vi "GDC Kom.vi"(6 "Befehl":T3, 8 "error in (no error)":errorcluster caption="Fehler (Eingang, kein Fehler)", 10 "Daten":string[](array[string]), 11 "Serielle Parameter":T2={"VISA resource name"="", "timeout"=10000, "baud rate"=9600, "data bits "=8, "stop bits "=10, "Enable Termination\nChar (T)"=TRUE, "termination char\n(0xA = '\\n' = LF) "=13} {"termination char\n(0xA = '\\n' = LF)" format="%.0x"; "stop bits" items=["1.0"=10, "1.5"=15, "2.0"=20]; "data bits" min=5 max=8 step=1}) -> (0 "error out":errorcluster caption="Fehler (Ausgang)", 1 "Status (alarm)":bool, 2 "Gas":string[](array[string]), 3 "Fehler":bool, 4 "Status":string, 5 "Konzentration":string, 7 "Konzentration 2":string)   [LabVIEW 2020, in "Linearisierung v2.lvlib" / "Gasteiler.lvlib" / "Horiba GDC.lvlib"]
uses:
  Horiba GDC.lvlib
  Aktion Befehl.ctl
  Serielle Parameter.ctl
  Stats.ctl
  Aktionen FGV Gasteiler Daten.ctl
  <vilib>/Instr/_visa.llb/VISA Configure Serial Port (Instr).vi
  Gasteiler.lvlib
panel:
  out "Status":T1
  out "Daten":string
  out "Befehl":string
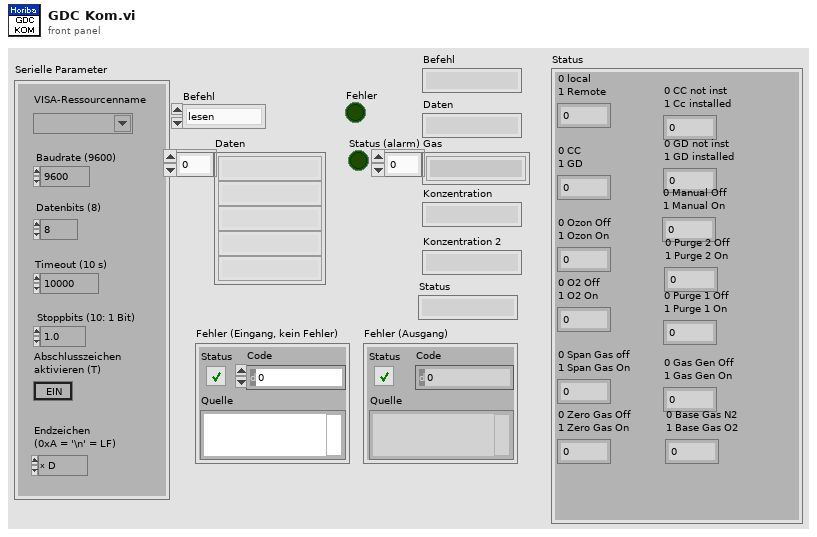
[diagram p1: front panel]
types:
  T1 = typedef "Linearisierung v2.lvlib/Gasteiler.lvlib/Horiba GDC.lvlib/Stats.ctl" = cluster{"0 local\n1 Remote":i16, "0 CC\n1 GD":i16, "0 Ozon Off\n1 Ozon On":i16, "0 O2 Off\n1 O2 On":i16, "0 Span Gas off\n1 Span Gas On ":i16, "0 Zero Gas Off\n1 Zero Gas On":i16, "0 CC not inst\n1 Cc installed":i16, "0 GD not inst\n1 GD installed":i16, "0 Manual Off\n1 Manual On":i16, "0 Purge 2 Off\n1 Purge 2 On":i16, "0 Purge 1 Off\n1 Purge 1 On":i16, "0 Gas Gen Off\n1 Gas Gen On":i16, "0 Base Gas N2\n1 Base Gas O2":i16}
  T2 = typedef "Linearisierung v2.lvlib/Gasteiler.lvlib/Horiba GDC.lvlib/Serielle Parameter.ctl" = cluster{"VISA resource name":refnum<visa-resource-name>, "timeout":u32, "baud rate":u32, "data bits ":u16, "stop bits ":u16, "Enable Termination\nChar (T)":bool, "termination char\n(0xA = '\\n' = LF) ":u8}
  T3 = typedef "Linearisierung v2.lvlib/Gasteiler.lvlib/Horiba GDC.lvlib/Aktion Befehl.ctl" = enum16{"lesen", "initialisieren", "Beenden", "Standby", "GD/CC", "Info", "Flow", "Alarm", "GD parameter", "GD point", "Durchfluss", "Spuelen1", "Spuelen1 On", "Spuelen1Off", "Spuelen2", "Ventil-Abfrage", "Reset"}
  T4 = typedef "Linearisierung v2.lvlib/Gasteiler.lvlib/Aktionen FGV Gasteiler Daten.ctl" = enum16{"lesen", "Gasteiler Daten", "Seriellen Param.", "MB-Endwert", "laden", "speichern", "Anforderung", "TCP", "Aufzeichnung Start"}
  T5 = typedef "AK-Schnittstelle.lvlib/AK Seriell.lvlib/Serielle Parameter.ctl" = cluster{"VISA resource name":refnum<visa-resource-name>, "baud rate":u32, "data bits":u16, "parity":u16, "stop bits":u16, "flow control":u16}
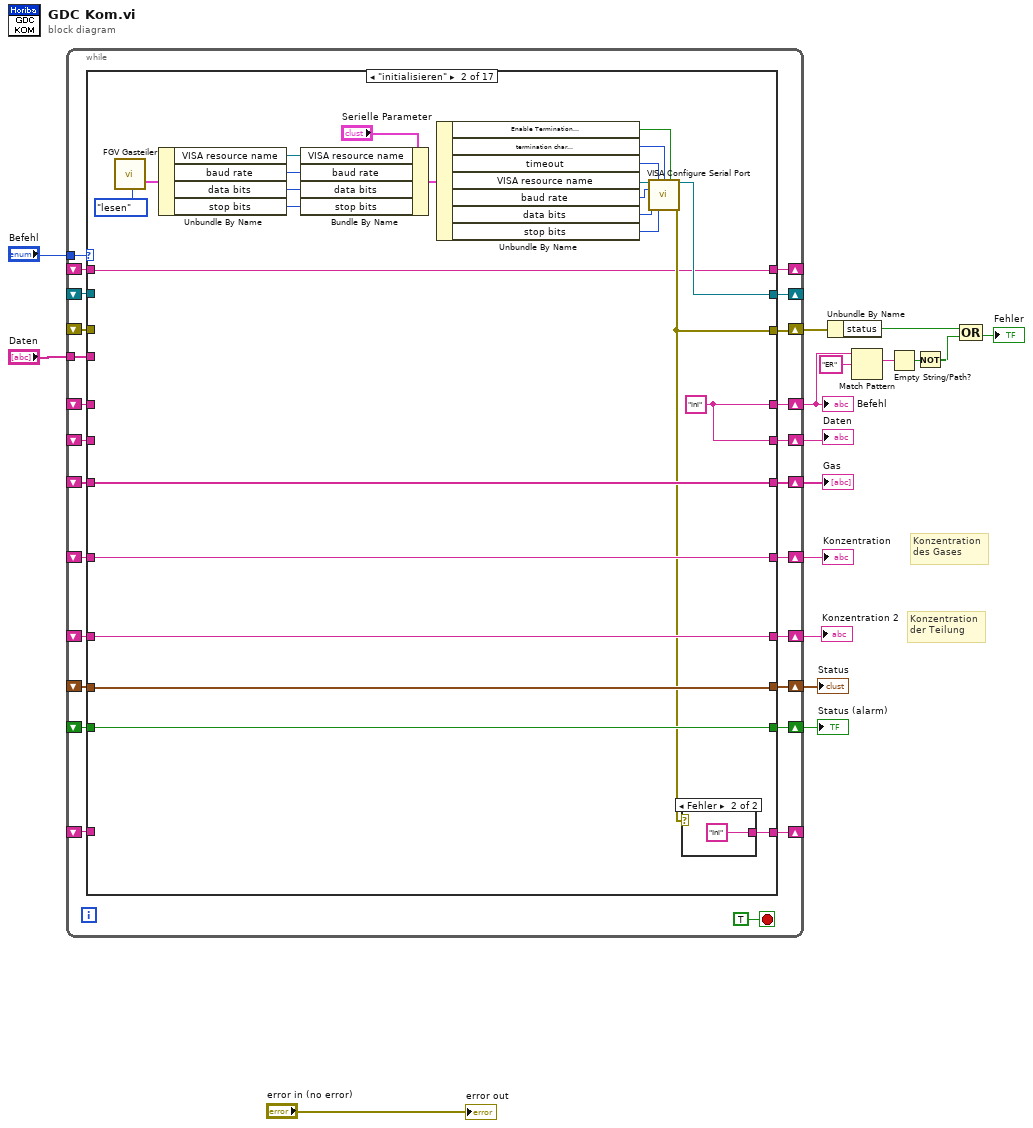
[diagram p0: block diagram]
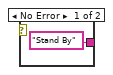
[diagram p3: hidden frame]
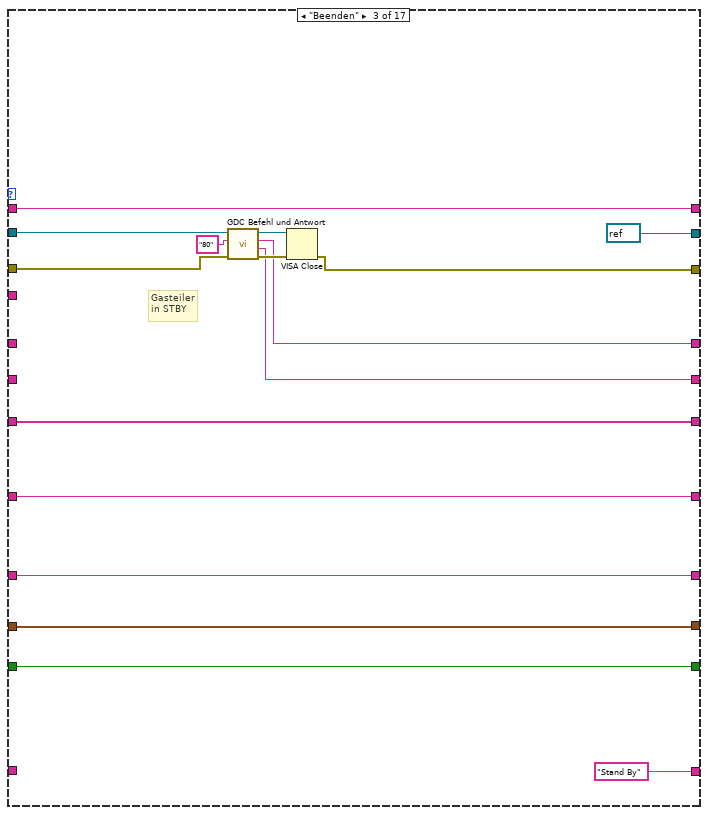
[diagram p4: hidden frame]
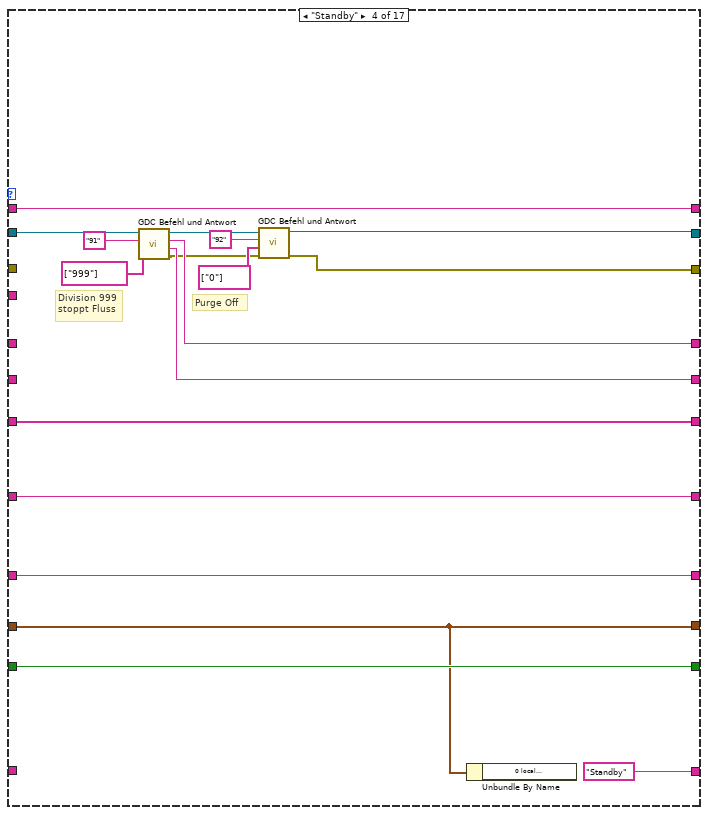
[diagram p5: hidden frame]
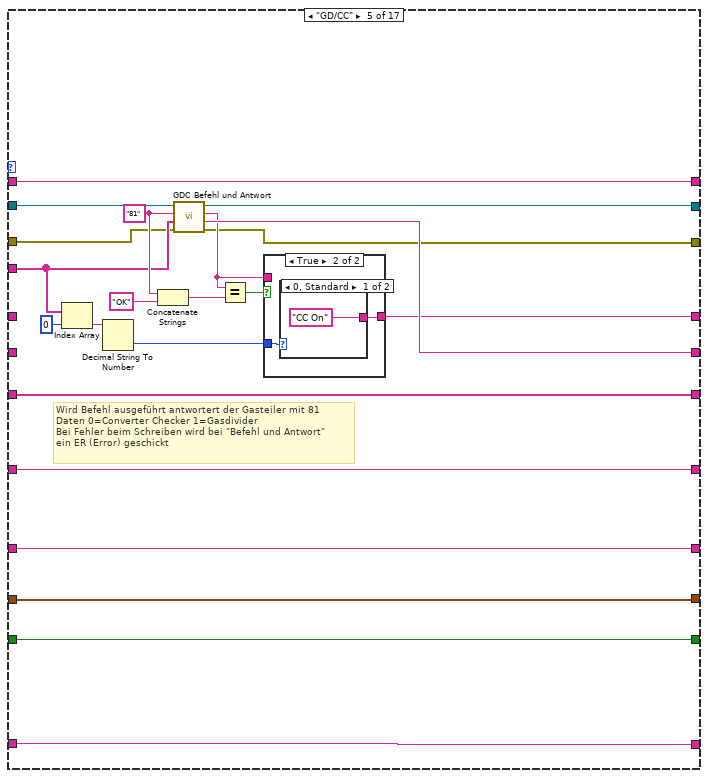
[diagram p6: hidden frame]
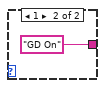
[diagram p8: hidden frame]
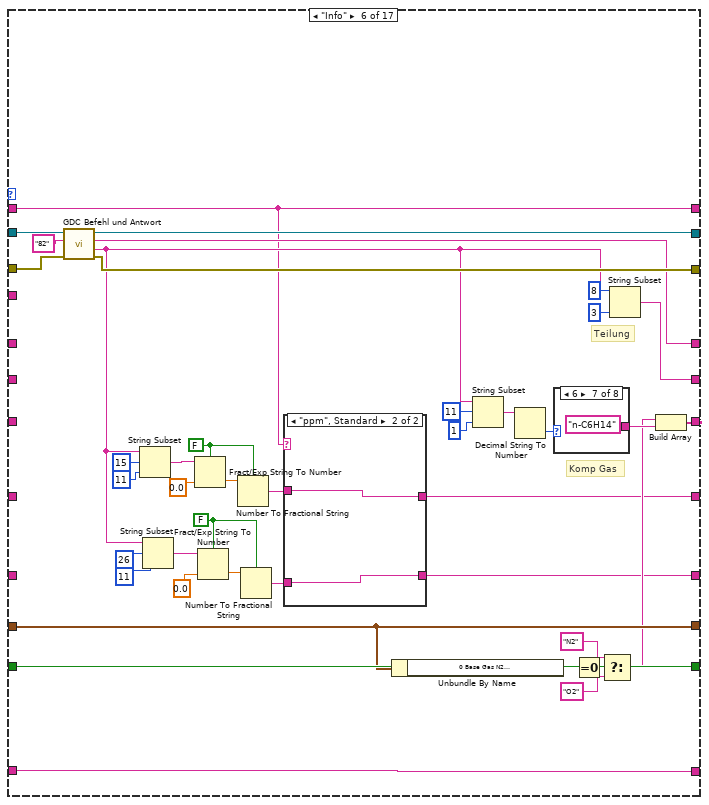
[diagram p9: hidden frame]
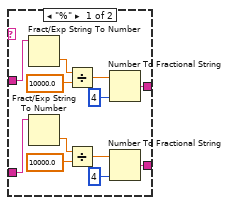
[diagram p10: hidden frame]
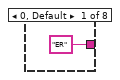
[diagram p11: hidden frame]
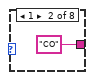
[diagram p12: hidden frame]
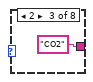
[diagram p13: hidden frame]
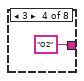
[diagram p14: hidden frame]
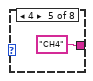
[diagram p15: hidden frame]
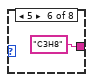
[diagram p16: hidden frame]
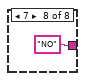
[diagram p17: hidden frame]
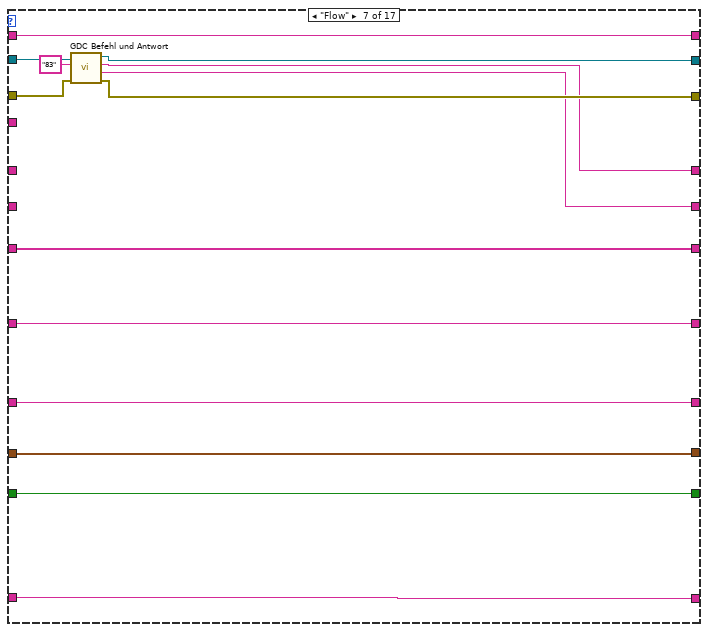
[diagram p18: hidden frame]
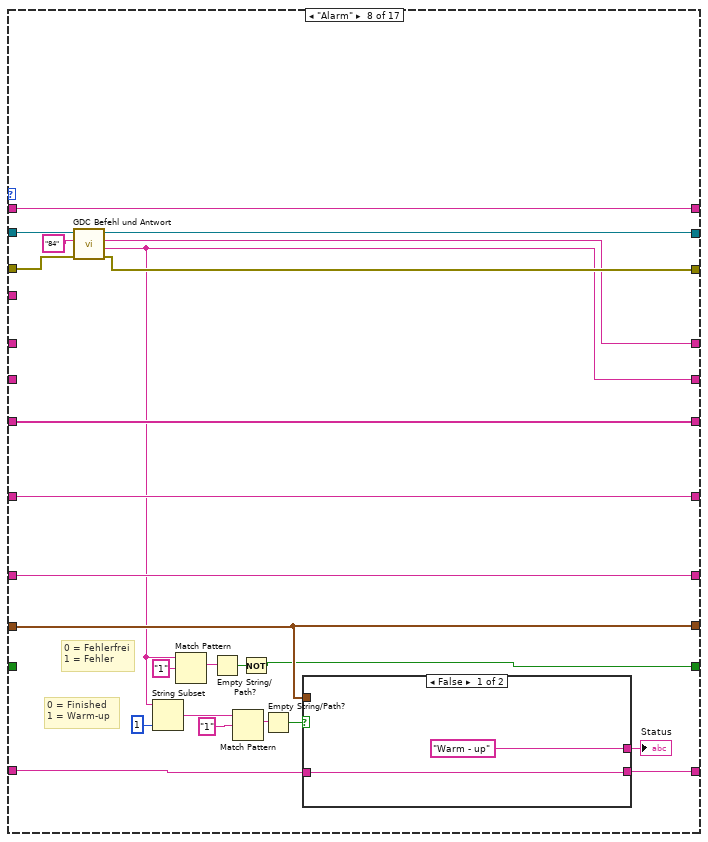
[diagram p19: hidden frame]
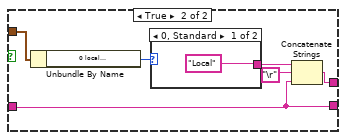
[diagram p20: hidden frame]
diagram:
  # "Konzentration\nder Teilung"
  # "Konzentration\ndes Gases"
  n1 = while {
    tunnel: "Befehl" -> [w41]
    shift-right: [w40] -> _
    shift-left: _ -> [w39]
    shift-right: [w38] -> w3
    shift-left: _ -> [w37]
    tunnel: "Daten" -> [w35]
    shift-right: [w36] -> w8
    shift-left: _ -> [w29]
    shift-right: [w34] -> w15
    shift-left: _ -> [w28]
    shift-right: [w33] -> w14
    shift-left: _ -> [w27]
    shift-right: [w32] -> w13
    shift-left: _ -> [w26]
    shift-right: [w31] -> w12
    shift-left: _ -> [w25]
    shift-right: [w30] -> w4
    shift-left: _ -> [w24]
    shift-right: [w23] -> w2
    shift-left: _ -> [w22]
    shift-right: [w20] -> _
    shift-left: _ -> [w21]
    shift-right: [w19] -> _
    shift-left: _ -> [w18]
    stop <- TRUE stop-if-true
    n2 = case shown="\"initialisieren\"" w41 {
      tunnel: [w53 w73 refnum<visa-resource-name> refnum ("VISA resource name out") w100 w135 w180 w209 w238 w285 w309 w371 w386 w401 w414 w425 w439 w453] -> w40
      tunnel: w39 -> [w53 _ w91 w114 w136 w182 w213 w242 w288 w334 w373 w388 w403 w417 w429 w441 w455]
      tunnel: [w52 w56 w95 w101 w124 w179 w210 w239 w284 w307 w370 w385 w400 w413 w424 w440 w452] -> w38
      tunnel: w37 -> [w52 _ w92 _ w125 w181 w211 w241 w287 w333 w372 w387 w402 w416 w428 w442 w454]
      tunnel: [w51 w72 w85 w112 w131 w158 w208 w232 w283 w308 w367 w383 w398 w412 w423 w438 w451] -> w36
      tunnel: w35 -> [_ _ _ _ w129 _ _ _ w257 w331 w368 _ _ w415 _ _ _]
      tunnel: [w50 w72 w84 w111 w134 w176 w207 w220 w282 w306 w366 w382 w397 w411 w422 w437 w461] -> w34
      tunnel: [w49 w71 w90 w110 w123 w154 w218 w222 w281 w302 w365 w381 w396 w410 w433 w447 w460] -> w33
      tunnel: [w48 w70 w89 w109 w122 w143 w217 w234 w261 w292 w364 w380 w395 w409 w432 w446 w459] -> w32
      tunnel: [w47 w69 w88 w108 w121 w142 w216 w233 w280 w291 w363 w379 w394 w408 w431 w445 w458] -> w31
      tunnel: [w46 w68 w87 w107 w120 w157 w215 w219 w279 w330 w362 w378 w393 w407 w430 w444 w457] -> w30
      tunnel: w29 -> [w51 _ _ _ _ _ _ _ _ _ _ _ _ _ _ _ _]
      tunnel: w28 -> [w50 _ _ _ _ _ _ _ _ _ _ _ _ _ _ _ w461]
      tunnel: w27 -> [w49 w71 w90 w110 w123 _ w218 w222 w281 _ w365 w381 w396 w410 w433 w447 w460]
      tunnel: w26 -> [w48 w70 w89 w109 w122 _ w217 w234 w261 _ w364 w380 w395 w409 w432 w446 w459]
      tunnel: w25 -> [w47 w69 w88 w108 w121 _ w216 w233 w280 _ w363 w379 w394 w408 w431 w445 w458]
      tunnel: w24 -> [w46 w68 w87 w107 w120 w157 w215 _ w279 w330 w362 w378 w393 w407 w430 w444 w457]
      tunnel: [w45 w58 w83 w99 w117 w149 w214 w223 w260 w296 w361 w377 w392 w406 w421 w436 w450] -> w23
      tunnel: w22 -> [w45 w58 w83 w99 w117 w149 w214 w223 w260 _ w361 w377 w392 w406 w421 w436 w450]
      tunnel: w21 -> [w44 _ _ _ w116 w155 w206 w226 _ _ _ _ _ _ w420 w435 _]
      tunnel: [w44 w57 "Stand By" "Standby" w116 w155 w206 w225 "Set" "CalGas" "Purge" "Purge" "Stand By" "Purge Air" w420 w435 "Stand By"] -> w20
      tunnel: [w43 w55 w81 w97 w115 w144 w205 w221 w254 w293 w359 w374 w389 w404 w419 w434 w448] -> w19
      tunnel: w18 -> [w43 w55 w81 w97 w115 w144 w205 w221 _ w293 w359 w374 w389 w404 w419 w434 w448]
      frame "lesen", Default {
      }
      frame "initialisieren" {
        w72 = "ini" ("Befehl")
        n3 = call "FGV Gasteiler.vi"("Aktionen"=Aktionen_FGV_Gasteiler_Daten."lesen") -> ("Serielle Parameter"=w65:T5)  [unwired: 11 in, 7 out]
        n4 = Unbundle By Name(w65) -> ("VISA resource name"=w59:refnum<visa-resource-name>, "baud rate"=w60:u32, "data bits"=w61:u16, "stop bits"=w62:u16)
        n5 = Bundle By Name(cluster="Serielle Parameter", "VISA resource name"=w59, "baud rate"=w60, "data bits"=w61, "stop bits"=w62) -> (w64:T2)
        n6 = Unbundle By Name(w64) -> ("Enable Termination\nChar (T)"=w67:bool, "termination char\n(0xA = '\\n' = LF)"=w66:u8, "timeout"=w78:u32, "VISA resource name"=w77:refnum<visa-resource-name>, "baud rate"=w76:u32, "data bits"=w75:u16, "stop bits"=w74:u16)
        n7 = call-poly "VISA Configure Serial Port"("VISA resource name"=w77, "timeout (10sec)"=w78, "termination char\n(0xA = '\\n' = LF)"=w66, "Enable Termination\nChar (T)"=w67, "baud rate (9600)"=w76, "data bits (8)"=w75, "stop bits (10: 1 bit)"=w74) -> ("VISA resource name out"=w73:refnum<visa-resource-name>, "error out"=w56:errorcluster)  [unwired: 7 in]
        n8 = case shown="Fehler" w56 {
          tunnel: ["Stand By" "Ini" ("Befehl")] -> w57
          frame No Error {
          }
          frame Error {
          }
        }
      }
      frame "Beenden" {
        # "Gasteiler\nin STBY"
        n9 = call "GDC Befehl und Antwort.vi"("error in (no error)"=w92, "Befehl"="80", "VISA-Ressourcenname"=w91) -> ("error out"=w93:errorcluster, "Daten"=w84:string, "Befehl"=w85:string, "VISA-Ressourcenname (Ausgang)"=w86:refnum<visa-resource-name>)  [unwired: 5 in]
        n10 = VISA Close(VISA resource name=w86, error in (no error)=w93) -> (error out=w95:errorcluster)
      }
      frame "Standby" {
        # "Purge Off"
        # "Division 999\nstoppt Fluss"
        n11 = call "GDC Befehl und Antwort.vi"("Daten"=string[] ["999"], "Befehl"="91", "VISA-Ressourcenname"=w114) -> ("error out"=w102:errorcluster, "Daten"=w111:string, "Befehl"=w112:string, "VISA-Ressourcenname (Ausgang)"=w103:refnum<visa-resource-name>)  [unwired: 5 in]
        n12 = call "GDC Befehl und Antwort.vi"("error in (no error)"=w102, "Daten"=string[] ["0"], "Befehl"="92", "VISA-Ressourcenname"=w103) -> ("error out"=w101:errorcluster, "VISA-Ressourcenname (Ausgang)"=w100:refnum<visa-resource-name>)  [unwired: 4 in, 2 out]
        n13 = Unbundle By Name(w99) -> ()  [unwired: 1 out]
      }
      frame "GD/CC" {
        w133 = "81" ("Befehl")
        # "Wird Befehl ausgeführt antwortert der Gasteiler mit 81\nDaten 0=Converter Checker 1=Gasdivider\nBei Fehler beim Schreiben wird bei \"Befehl und Antwort\"\nein ER (Error) geschickt"
        n14 = Index Array(array=w129, index=0 ("Index")) -> (element=w127:string)
        n15 = Decimal String To Number(string=w127) -> (number=w126:i32)  [unwired: 2 in, 1 out]
        n16 = Concatenate Strings(w133, "OK" ("String")) -> (w119:string)
        n17 = call "GDC Befehl und Antwort.vi"("error in (no error)"=w125, "Daten"=w129, "Befehl"=w133, "VISA-Ressourcenname"=w136) -> ("error out"=w124:errorcluster, "Daten"=w134:string, "Befehl"=w130:string, "VISA-Ressourcenname (Ausgang)"=w135:refnum<visa-resource-name>)  [unwired: 4 in]
        n18 = Equal?(x=w130, y=w119) -> (x = y?=w132:bool)
        n19 = case shown="True" w132 {
          tunnel: [w137 w138] -> w131
          tunnel: w130 -> [w137 _]
          tunnel: w126 -> [_ w139]
          frame False {
          }
          frame True {
            n20 = case shown="0, Standard" w139 {
              tunnel: ["CC On" ("Befehl") "GD On" ("Befehl")] -> w138
              frame 0, Default {
              }
              frame 1 {
              }
            }
          }
        }
      }
      frame "Info" {
        w165 = FALSE ("Systemdezimalzeichen verwenden (T)")
        w166 = FALSE ("Systemdezimalzeichen verwenden (T)")
        # "Komp Gas"
        # "Teilung"
        n21 = call "GDC Befehl und Antwort.vi"("error in (no error)"=w181, "Befehl"="82", "VISA-Ressourcenname"=w182) -> ("error out"=w179:errorcluster, "Daten"=w159:string, "Befehl"=w158:string, "VISA-Ressourcenname (Ausgang)"=w180:refnum<visa-resource-name>)  [unwired: 5 in]
        n22 = String Subset(string=w159, offset (0)=15 ("Offset (0)"), length (rest)=11 ("Länge (Rest)")) -> (substring=w169:string)
        n23 = String Subset(string=w159, offset (0)=26 ("Offset (0)"), length (rest)=11 ("Länge (Rest)")) -> (substring=w162:string)
        n24 = Fract/Exp String To Number(use system decimal point (T)=w166, string=w169, default (0 dbl)=sgl 0.0 ("Standard (0 DBL)")) -> (number=w167:sgl)  [unwired: 1 in, 1 out]
        n25 = Fract/Exp String To Number(use system decimal point (T)=w165, string=w162, default (0 dbl)=sgl 0.0 ("Standard (0 DBL)")) -> (number=w164:sgl)  [unwired: 1 in, 1 out]
        n26 = Number To Fractional String(use system decimal point (T)=w166, number=w167) -> (F-format string=w146:string)  [unwired: 2 in]
        n27 = Number To Fractional String(use system decimal point (T)=w165, number=w164) -> (F-format string=w145:string)  [unwired: 2 in]
        n28 = case shown="\"ppm\", Standard" w144 {
          tunnel: [w190 w195] -> w142
          tunnel: [w185 w196] -> w143
          tunnel: w146 -> [w184 w196]
          tunnel: w145 -> [w183 w195]
          frame "%" {
            n29 = Fract/Exp String To Number(string=w184) -> (number=w187:dbl)  [unwired: 3 in, 1 out]
            n30 = Fract/Exp String To Number(string=w183) -> (number=w193:dbl)  [unwired: 3 in, 1 out]
            n31 = Divide(x=w187, y=10000.0) -> (x/y=w188:dbl)
            n32 = Divide(x=w193, y=10000.0) -> (x/y=w192:dbl)
            n33 = Number To Fractional String(number=w188, precision (6)=i16 4 ("Genauigkeit (6)")) -> (F-format string=w185:string)  [unwired: 2 in]
            n34 = Number To Fractional String(number=w192, precision (6)=i16 4 ("Genauigkeit (6)")) -> (F-format string=w190:string)  [unwired: 2 in]
          }
          frame "ppm", Default {
          }
        }
        n35 = Unbundle By Name(w149) -> ("0 Base Gas N2\n1 Base Gas O2"=w153:i16)
        n36 = String Subset(string=w159, offset (0)=11 ("Offset (0)"), length (rest)=1 ("Länge (Rest)")) -> (substring=w173:string)
        n37 = Decimal String To Number(string=w173) -> (number=w172:i32)  [unwired: 2 in, 1 out]
        n38 = case shown="6" w172 {
          tunnel: ["ER" ("Befehl") "CO" ("Befehl") "CO2" ("Befehl") "O2" ("Befehl") "CH4" ("Befehl") "C3H8" ("Befehl") "n-C6H14" ("Befehl") "NO" ("Befehl")] -> w148
          frame 0, Default {
          }
          frame 1 {
          }
          frame 2 {
          }
          frame 3 {
          }
          frame 4 {
          }
          frame 5 {
          }
          frame 6 {
          }
          frame 7 {
          }
        }
        n39 = Equal To 0?(x=w153) -> (x = 0?=w151:bool)
        n40 = Select(t="N2", s=w151, f="O2") -> (s? t:f=w147:string)
        n41 = String Subset(string=w159, offset (0)=8 ("Offset (0)"), length (rest)=3 ("Länge (Rest)")) -> (substring=w176:string)
        n42 = Build Array(w147, w148) -> (w154:string[])
      }
      frame "Flow" {
        n43 = call "GDC Befehl und Antwort.vi"("error in (no error)"=w211, "Befehl"="83", "VISA-Ressourcenname"=w213) -> ("error out"=w210:errorcluster, "Daten"=w207:string, "Befehl"=w208:string, "VISA-Ressourcenname (Ausgang)"=w209:refnum<visa-resource-name>)  [unwired: 5 in]
      }
      frame "Alarm" {
        # "0 = Finished\n1 = Warm-up"
        # "0 = Fehlerfrei\n1 = Fehler"
        n44 = call "GDC Befehl und Antwort.vi"("error in (no error)"=w241, "Befehl"="84", "VISA-Ressourcenname"=w242) -> ("error out"=w239:errorcluster, "Daten"=w220:string, "Befehl"=w232:string, "VISA-Ressourcenname (Ausgang)"=w238:refnum<visa-resource-name>)  [unwired: 5 in]
        n45 = String Subset(string=w220, length (rest)=1 ("Länge (Rest)")) -> (substring=w228:string)  [unwired: 1 in]
        n46 = Match Pattern(string=w220, regular expression="1" ("Regulärer Ausdruck")) -> (match substring=w236:string)  [unwired: 1 in, 3 out]
        n47 = Empty String/Path?(string/path=w236) -> (empty?=w235:bool)
        n48 = Match Pattern(string=w228, regular expression="1" ("Regulärer Ausdruck")) -> (match substring=w230:string)  [unwired: 1 in, 3 out]
        n49 = Not(x=w235) -> (.not. x?=w219:bool)
        n50 = Empty String/Path?(string/path=w230) -> (empty?=w227:bool)
        n51 = case shown="False" w227 {
          tunnel: w223 -> [_ w250]
          tunnel: ["Warm - up" w248] -> w224
          tunnel: w226 -> [w243 w246]
          tunnel: [w243 w246] -> w225
          frame False {
          }
          frame True {
            n52 = Unbundle By Name(w250) -> ("0 local\n1 Remote"=w249:i16)
            n53 = case shown="0, Standard" w249 {
              tunnel: ["Local" ("Regulärer Ausdruck") "Remote" ("Regulärer Ausdruck")] -> w247
              frame 0, Default {
              }
              frame 1 {
              }
            }
            n54 = Concatenate Strings(w247, "\r", w246) -> (w248:string)
          }
        }
        "Status" <- w224
      }
      frame "GD parameter" {
        # "#GenauSysFix"
        # "Befehl:\n90\nx - 1-7 für Komp Gas\nx - 1-2 für Träger Gas\nxxx - Teilung (z.B. 001 -500)\nxxxxxxxxxxx - für Konzentration in ppm z.B. +1.23456E+09"
        n55 = Array Size(array=w257) -> (size(s)=w258:i32)
        n56 = Decrement(x=w258) -> (x-1=w256:i32)
        n57 = Delete From Array(array=w257, index=w256) -> (deleted portion=w254:string, array with subset deleted=w255:string[])  [unwired: 1 in]
        n58 = Index Array(array=w255, index=3 ("Index")) -> (element=w272:string)
        n59 = Fract/Exp String To Number(use system decimal point (T)=FALSE ("Systemdezimalzeichen verwenden (T)"), string=w272, default (0 dbl)=sgl 0.0 ("Standard (0 I32)")) -> (number=w276:sgl)  [unwired: 1 in, 1 out]
        n60 = Number To Exponential String(number=w276, precision (6)=i16 4 ("Genauigkeit (6)"), 1:FALSE ("Systemdezimalzeichen verwenden (T)")) -> (E-format string=w266:string)  [unwired: 1 in]
        n61 = String Subset(string=w266, length (rest)=8 ("Länge (Rest)")) -> (substring=w263:string)  [unwired: 1 in]
        n62 = String Subset(string=w266, offset (0)=8 ("Offset (0)")) -> (substring=w267:string)  [unwired: 1 in]
        n63 = Concatenate Strings(w263, "0" ("String"), w267) -> (w265:string)
        n64 = Concatenate Strings("+" ("String"), w265) -> (w271:string)
        n65 = Replace Array Subset(array=w255, new element=w271, index=3 ("Index")) -> (w273:string[])
        n66 = call "GDC Befehl und Antwort.vi"("error in (no error)"=w287, "Daten"=w273, "Befehl"="90", "VISA-Ressourcenname"=w288) -> ("error out"=w284:errorcluster, "Daten"=w282:string, "Befehl"=w283:string, "VISA-Ressourcenname (Ausgang)"=w285:refnum<visa-resource-name>)  [unwired: 4 in]
      }
      frame "GD point" {
        w317 = FALSE ("Systemdezimalzeichen verwenden (T)")
        w318 = FALSE ("Systemdezimalzeichen verwenden (T)")
        # "Konzentration des \naktuellen Punkts\nund Konzentration \ndes Gases???"
        # "Komp Gas"
        # "Teilung"
        # "Befehl\n91\nxxx - Teilungsstufe z.B. 192"
        n67 = call "GDC Befehl und Antwort.vi"("error in (no error)"=w333, "Daten"=w331, "Befehl"="91", "VISA-Ressourcenname"=w334) -> ("error out"=w290:errorcluster, "VISA-Ressourcenname (Ausgang)"=w310:refnum<visa-resource-name>)  [unwired: 4 in, 2 out]
        n68 = flat-sequence {
          tunnel: w290 -> [w335]
          tunnel: [w335] -> w289
          frame #0 {
            n69 = Wait (ms)(milliseconds to wait=u32 500 ("Zu wartende ms")) -> ()  [unwired: 1 out]
          }
        }
        n70 = call "GDC Befehl und Antwort.vi"("error in (no error)"=w289, "Befehl"="82", "VISA-Ressourcenname"=w310) -> ("error out"=w307:errorcluster, "Daten"=w304:string, "Befehl"=w308:string, "VISA-Ressourcenname (Ausgang)"=w309:refnum<visa-resource-name>)  [unwired: 5 in]
        n71 = call "Hex String.vi"("Eingabe String"=w304) -> ("Status"=w296:T1)  [unwired: 10 in]
        n72 = String Subset(string=w304, offset (0)=26 ("Offset (0)"), length (rest)=11 ("Länge (Rest)")) -> (substring=w314:string)
        n73 = String Subset(string=w304, offset (0)=15 ("Offset (0)"), length (rest)=11 ("Länge (Rest)")) -> (substring=w321:string)
        n74 = Unbundle By Name(w296) -> ("0 Base Gas N2\n1 Base Gas O2"=w301:i16)
        n75 = Fract/Exp String To Number(use system decimal point (T)=w317, string=w314, default (0 dbl)=sgl 0.0 ("Standard (0 DBL)")) -> (number=w316:sgl)  [unwired: 1 in, 1 out]
        n76 = Fract/Exp String To Number(use system decimal point (T)=w318, string=w321, default (0 dbl)=sgl 0.0 ("Standard (0 DBL)")) -> (number=w319:sgl)  [unwired: 1 in, 1 out]
        n77 = Number To Fractional String(use system decimal point (T)=w317, number=w316) -> (F-format string=w294:string)  [unwired: 2 in]
        n78 = Number To Fractional String(use system decimal point (T)=w318, number=w319) -> (F-format string=w295:string)  [unwired: 2 in]
        n79 = case shown="\"ppm\", Standard" w293 {
          tunnel: [w344 w349] -> w291
          tunnel: [w339 w350] -> w292
          tunnel: w295 -> [w338 w350]
          tunnel: w294 -> [w337 w349]
          frame "%" {
            n80 = Fract/Exp String To Number(string=w338) -> (number=w341:dbl)  [unwired: 3 in, 1 out]
            n81 = Fract/Exp String To Number(string=w337) -> (number=w347:dbl)  [unwired: 3 in, 1 out]
            n82 = Divide(x=w341, y=10000.0) -> (x/y=w342:dbl)
            n83 = Divide(x=w347, y=10000.0) -> (x/y=w346:dbl)
            n84 = Number To Fractional String(number=w342, precision (6)=i16 4 ("Genauigkeit (6)")) -> (F-format string=w339:string)  [unwired: 2 in]
            n85 = Number To Fractional String(number=w346, precision (6)=i16 4 ("Genauigkeit (6)")) -> (F-format string=w344:string)  [unwired: 2 in]
          }
          frame "ppm", Default {
          }
        }
        n86 = String Subset(string=w304, offset (0)=11 ("Offset (0)"), length (rest)=1 ("Länge (Rest)")) -> (substring=w325:string)
        n87 = Decimal String To Number(string=w325) -> (number=w324:i32)  [unwired: 2 in, 1 out]
        n88 = Equal To 0?(x=w301) -> (x = 0?=w299:bool)
        n89 = Select(t="N2", s=w299, f="O2") -> (s? t:f=w297:string)
        n90 = case shown="0, Standard" w324 {
          tunnel: ["ER" ("Befehl") "CO" ("Befehl") "CO2" ("Befehl") "O2" ("Befehl") "CH4" ("Befehl") "C3H8" ("Befehl") "n-C6H14" ("Befehl") "NO" ("Befehl")] -> w305
          frame 0, Default {
          }
          frame 1 {
          }
          frame 2 {
          }
          frame 3 {
          }
          frame 4 {
          }
          frame 5 {
          }
          frame 6 {
          }
          frame 7 {
          }
        }
        n91 = String Subset(string=w304, offset (0)=8 ("Offset (0)"), length (rest)=3 ("Länge (Rest)")) -> (substring=w306:string)
        n92 = Build Array(w297, w305) -> (w302:string[])
      }
      frame "Spuelen1" {
        # "Purge 1 für GD\n0 = Reset\n1 = Purge"
        n93 = call "GDC Befehl und Antwort.vi"("error in (no error)"=w372, "Daten"=w368, "Befehl"="92", "VISA-Ressourcenname"=w373) -> ("error out"=w370:errorcluster, "Daten"=w366:string, "Befehl"=w367:string, "VISA-Ressourcenname (Ausgang)"=w371:refnum<visa-resource-name>)  [unwired: 4 in]
      }
      frame "Spuelen1 On" {
        # "Purge 1 für GD\n0 = Reset\n1 = Purge"
        n94 = call "GDC Befehl und Antwort.vi"("error in (no error)"=w387, "Daten"=string[] ["1"], "Befehl"="92", "VISA-Ressourcenname"=w388) -> ("error out"=w385:errorcluster, "Daten"=w382:string, "Befehl"=w383:string, "VISA-Ressourcenname (Ausgang)"=w386:refnum<visa-resource-name>)  [unwired: 4 in]
      }
      frame "Spuelen1Off" {
        # "Purge 1 für GD\n0 = Reset\n1 = Purge"
        n95 = call "GDC Befehl und Antwort.vi"("error in (no error)"=w402, "Daten"=string[] ["0"], "Befehl"="92", "VISA-Ressourcenname"=w403) -> ("error out"=w400:errorcluster, "Daten"=w397:string, "Befehl"=w398:string, "VISA-Ressourcenname (Ausgang)"=w401:refnum<visa-resource-name>)  [unwired: 4 in]
      }
      frame "Spuelen2" {
        # "Purge 2 für GD\n0 = Reset\n1 = Purge"
        n96 = call "GDC Befehl und Antwort.vi"("error in (no error)"=w416, "Daten"=w415, "Befehl"="93", "VISA-Ressourcenname"=w417) -> ("error out"=w413:errorcluster, "Daten"=w411:string, "Befehl"=w412:string, "VISA-Ressourcenname (Ausgang)"=w414:refnum<visa-resource-name>)  [unwired: 4 in]
      }
      frame "Durchfluss" {
        # "NO Konz"
        # "Span Gas"
        # "Zero Gas"
        n97 = call "GDC Befehl und Antwort.vi"("error in (no error)"=w428, "Daten"=string[] ["0000", "4000", "0000000000"], "Befehl"="BD", "VISA-Ressourcenname"=w429) -> ("error out"=w424:errorcluster, "Daten"=w422:string, "Befehl"=w423:string, "VISA-Ressourcenname (Ausgang)"=w425:refnum<visa-resource-name>)  [unwired: 4 in]
      }
      frame "Ventil-Abfrage" {
        n98 = call "GDC Befehl und Antwort.vi"("error in (no error)"=w442, "Befehl"="B7", "VISA-Ressourcenname"=w441) -> ("error out"=w440:errorcluster, "Daten"=w437:string, "Befehl"=w438:string, "VISA-Ressourcenname (Ausgang)"=w439:refnum<visa-resource-name>)  [unwired: 5 in]
      }
      frame "Reset" {
        n99 = call "GDC Befehl und Antwort.vi"("error in (no error)"=w454, "Befehl"="80", "VISA-Ressourcenname"=w455) -> ("error out"=w452:errorcluster, "Befehl"=w451:string, "VISA-Ressourcenname (Ausgang)"=w453:refnum<visa-resource-name>)  [unwired: 5 in, 1 out]
      }
    }
  }
  "Befehl" <- w8
  "Daten" <- w15
  "Gas" <- w14
  "Konzentration" <- w13
  "Konzentration 2" <- w12
  "Status (alarm)" <- w4
  "Status" <- w2
  n100 = Unbundle By Name(w3) -> ("status"=w11:bool)
  n101 = Match Pattern(string=w8, regular expression="ER" ("Regulärer Ausdruck")) -> (match substring=w6:string)  [unwired: 1 in, 3 out]
  n102 = Empty String/Path?(string/path=w6) -> (empty?=w7:bool)
  n103 = Not(x=w7) -> (.not. x?=w5:bool)
  n104 = Compound Arithmetic op=OR ("Mehrfacharithmetik")(w11, w5) -> (→"Fehler":bool)
  "error out" <- "error in (no error)"
